vi "Read Transformation Matrix.vi"(8 "error in (no error)":errorcluster, 11 "Transform in":refnum<class "Transform.lvclass">) -> (0 "error out":errorcluster, 2 "Real Matrix":T1, 3 "Transform out":refnum<class "Transform.lvclass">)   [LabVIEW 2019, in "Transform.lvclass"]
uses:
  Transform.lvclass
  <vilib>/Analysis/Matrix/Datatypes/RealMatrix.ctl
  Transform.lvclass/Transform.ctl
  <vilib>/Analysis/Matrix/NI_Matrix.lvlib
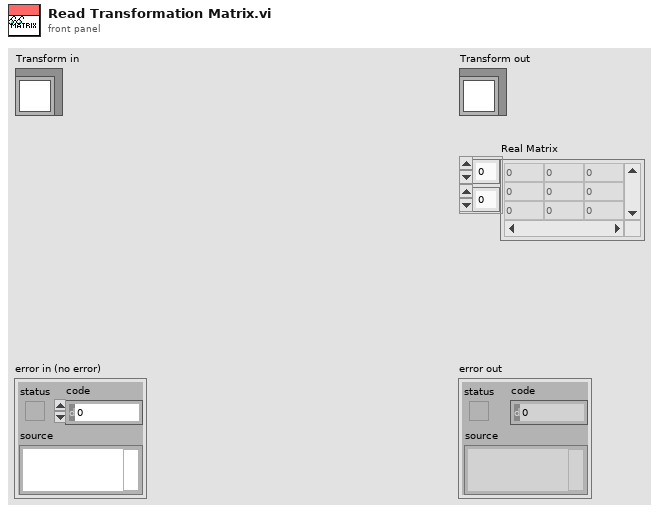
[diagram p1: front panel]
types:
  T1 = typedef "NI_Matrix.lvlib/RealMatrix.ctl" = dbl[][]
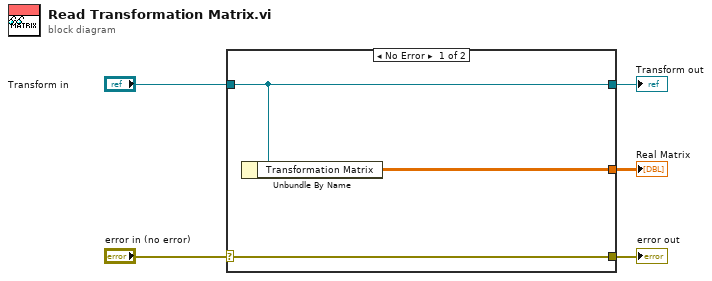
[diagram p0: block diagram]
diagram:
  n1 = case shown="No Error" "error in (no error)" {
    selector: "error in (no error)" -> [w8 w9]
    tunnel: [w8 w9] -> w4
    tunnel: [w7 w10] -> w2
    tunnel: "Transform in" -> [w7 w10]
    tunnel: [w6 _] -> w1
    frame No Error {
      n2 = Unbundle By Name(w7) -> ("Transformation Matrix"=w6:T1)
    }
    frame Error {
    }
  }
  "error out" <- w4
  "Transform out" <- w2
  "Real Matrix" <- w1
